vi "ALL VData Measurement.vi"(0 "VISA resource name":refnum<visa-resource-name>="DSOS404", 5 "txt path":string="D:\\TekScope\\DSOS404", 9 "TimeStamp":string="201711091702DSOS404", 11 "error in":errorcluster, 12 "Channel State":cluster{bool, bool, bool, bool}={TRUE, FALSE, FALSE, FALSE}) -> (4 "VISA resource name out":refnum<visa-resource-name>="DSOS404", 10 "Array":T1(array[cluster]), 15 "error out":errorcluster={"status"=TRUE, "code"=-1073807343, "source"="VISA Write in Open Channel.vi->ALL Data Measurement.vi"})   [LabVIEW 2018]
panel:
  out "concatenated string":string="AMP:\r\n0\r\n0\r\n0\r\n0\r\n\r\nFALL:\r\n0\r\n0\r\n0\r\n0\r\n\r\nMAX:\r\n0\r\n0\r\n0\r\n0\r\n\r\nPWI:\r\n0\r\n0\r\n0\r\n0\r\n\r\nRISE:\r\n0\r\n0\r\n0\r\n0\r\n"
  # "CH1"
  # "CH2"
  # "CH3"
  # "CH4"
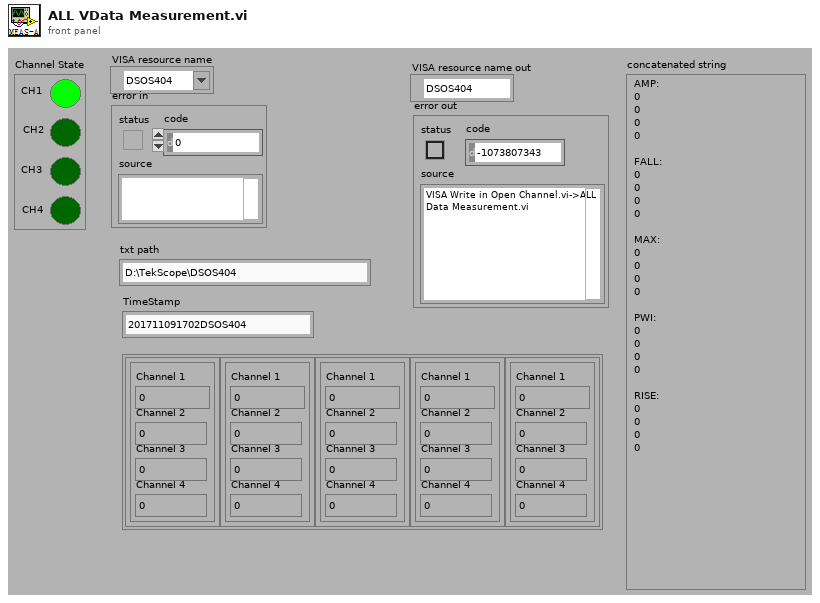
[diagram p1: front panel]
types:
  T1 = cluster{cluster{"Channel 1":dbl, "Channel 2":dbl, "Channel 3":dbl, "Channel 4":dbl}}[]
  T2 = cluster{"Channel 1":dbl, "Channel 2":dbl, "Channel 3":dbl, "Channel 4":dbl}
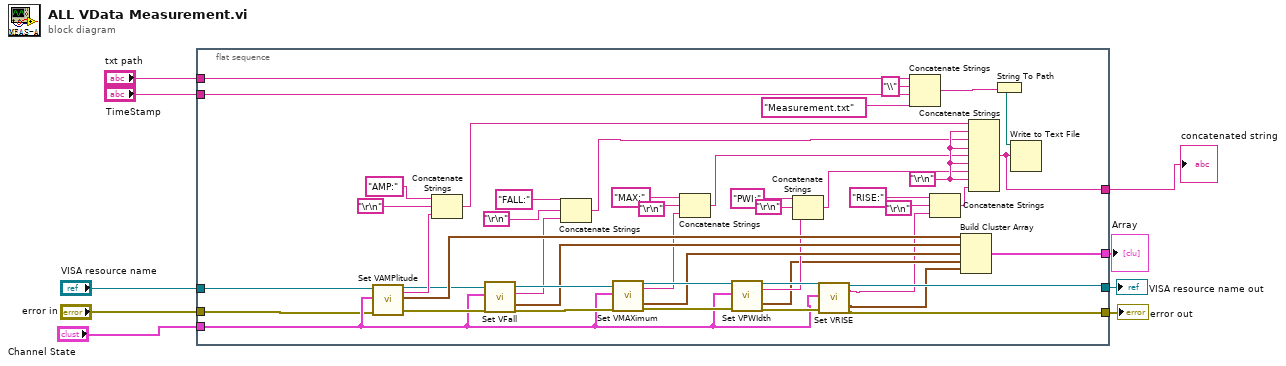
[diagram p0: block diagram]
diagram:
  n1 = flat-sequence {
    tunnel: [w56] -> w3
    tunnel: [w24] -> w6
    tunnel: [w21] -> w7
    tunnel: "TimeStamp" -> [w53]
    tunnel: "txt path" -> [w54]
    tunnel: "error in" -> [w10]
    tunnel: "VISA resource name" -> [w11]
    tunnel: "Channel State" -> [w20]
    tunnel: [w31] -> w1
    frame #0 {
      w49 = "\r\n"
      n2 = call "Set VAMPlitude.vi"("VISA resource name"=w11, "cluster"=w20, "error in (no error)"=w10) -> ("VISA resource name out"=w30:refnum<visa-resource-name>, "concatenated string"=w52:string, 18:w50:T2, "error out"=w28:errorcluster)  [unwired: 13 in]
      n3 = Concatenate Strings("AMP:" ("time format string (%c)"), "\r\n", w52) -> (w39:string)
      n4 = call "Set VFall.vi"("VISA resource name"=w30, "cluster"=w20, "error in (no error)"=w28) -> ("VISA resource name out"=w29:refnum<visa-resource-name>, "concatenated string"=w19:string, 18:w18:T2, "error out"=w27:errorcluster)  [unwired: 13 in]
      n5 = Concatenate Strings("FALL:" ("time format string (%c)"), "\r\n", w19) -> (w40:string)
      n6 = call "Set VMAXimum.vi"("VISA resource name"=w29, "cluster"=w20, "error in (no error)"=w27) -> ("VISA resource name out"=w23:refnum<visa-resource-name>, "concatenated string"=w17:string, 18:w16:T2, "error out"=w26:errorcluster)  [unwired: 13 in]
      n7 = Concatenate Strings("MAX:" ("time format string (%c)"), "\r\n", w17) -> (w41:string)
      n8 = call "Set VPWIdth.vi"("VISA resource name"=w23, "cluster"=w20, "error in (no error)"=w26) -> ("VISA resource name out"=w22:refnum<visa-resource-name>, "concatenated string"=w15:string, 18:w14:T2, "error out"=w25:errorcluster)  [unwired: 13 in]
      n9 = Concatenate Strings("PWI:" ("time format string (%c)"), "\r\n", w15) -> (w43:string)
      n10 = call "Set VRISE.vi"("VISA resource name"=w22, "cluster"=w20, "error in (no error)"=w25) -> ("VISA resource name out"=w21:refnum<visa-resource-name>, "concatenated string"=w13:string, 18:w12:T2, "error out"=w24:errorcluster)  [unwired: 13 in]
      n11 = Concatenate Strings(w54, "\\" ("string"), w53, "Measurement.txt" ("string")) -> (w33:string)
      n12 = Concatenate Strings("RISE:" ("time format string (%c)"), "\r\n", w13) -> (w42:string)
      n13 = Build Cluster Array(w50, w18, w16, w14, w12) -> (w56:T1)
      n14 = Concatenate Strings(w39, w49, w40, w49, w41, w49, w43, w49, w42) -> (w31:string)
      n15 = String To Path(string=w33) -> (path=w32:path)
      n16 = Write to Text File(file (use dialog)=w32, text=w31) -> ()  [unwired: 2 in, 3 out]
    }
  }
  "VISA resource name out" <- w7
  "error out" <- w6
  "Array" <- w3
  "concatenated string" <- w1
